vi "OEE_MAIN_set_default_reference.vi"(7 "all_config_info":T1, 8 "error_in":errorcluster, 11 "reference_selector":refnum<vi>) -> (0 "error_out":errorcluster, 3 "Default reference ok?":bool)   [LabVIEW 2019]
uses:
  ini/typedef/OEE_all_config_info.ctl
  ini/typedef/OEE_main_ini_file.ctl
  queues/typedef/OEE_queue_refnums.ctl
  queues/typedef/OEE_MAIN_queue_element.ctl
  OEE_MAIN_sequence_state.ctl
  queues/typedef/OEE_SCREEN_1_queue_element.ctl
  SCREEN_1/OEE_SCREEN_1_sequence_state.ctl
  queues/typedef/OEE_SCREEN_2_queue_element.ctl
  SCREEN_2/OEE_SCREEN_2_sequence_state.ctl
  queues/typedef/OEE_PULSE_queue_element.ctl
  PULSE/OEE_PULSE_sequence_state.ctl
  queues/typedef/OEE_GRAPH_TOGGLE_TIMER_queue_element.ctl
  SCREEN_2/GRAPH_TOGGLE_TIMER/OEE_GRAPH_TOGGLE_TIMER_sequence_state.ctl
  FGV/reference_selector/FGV_OEE_reference_selector.ctl
  _misc/AULocalize/SubVIs/Get Localized Phrase Compact Interface 0D.vi
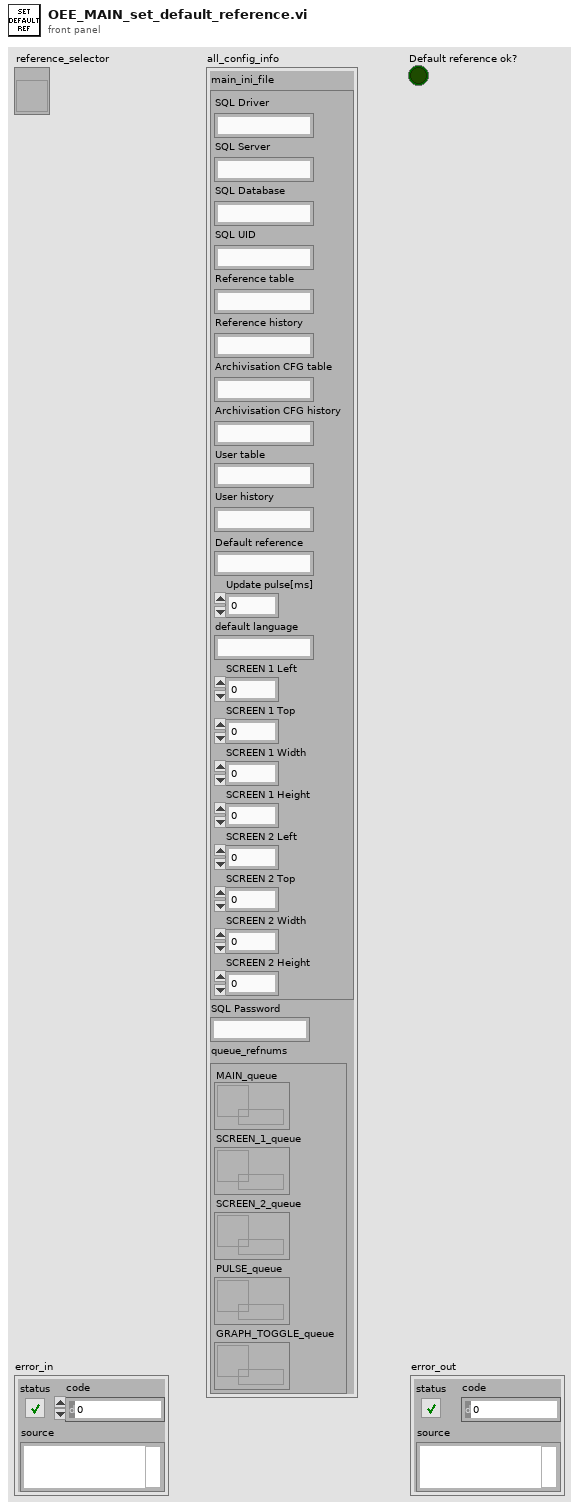
[diagram p1: front panel]
types:
  T1 = typedef "OEE_all_config_info.ctl" = cluster{"main_ini_file":T2, "SQL Password":string, "queue_refnums":T3}
  T2 = typedef "OEE_main_ini_file.ctl" = cluster{"SQL Driver":string, "SQL Server":string, "SQL Database":string, "SQL UID":string, "Reference table":string, "Reference history":string, "Archivisation CFG table":string, "Archivisation CFG history":string, "User table":string, "User history":string, "Default reference":string, "Update pulse[ms]":i32, "default language":string, "SCREEN 1 Left":i16, "SCREEN 1 Top":i16, "SCREEN 1 Width":i16, "SCREEN 1 Height":i16, "SCREEN 2 Left":i16, "SCREEN 2 Top":i16, "SCREEN 2 Width":i16, "SCREEN 2 Height":i16}
  T3 = typedef "OEE_queue_refnums.ctl" = cluster{"MAIN_queue":refnum<queue>, "SCREEN_1_queue":refnum<queue>, "SCREEN_2_queue":refnum<queue>, "PULSE_queue":refnum<queue>, "GRAPH_TOGGLE_queue":refnum<queue>}
  T4 = typedef "FGV_OEE_reference_selector.ctl" = enum16{"initialize", "set_values", "enable", "disable", "disable_gray", "get_reference_list", "get_active_reference"}
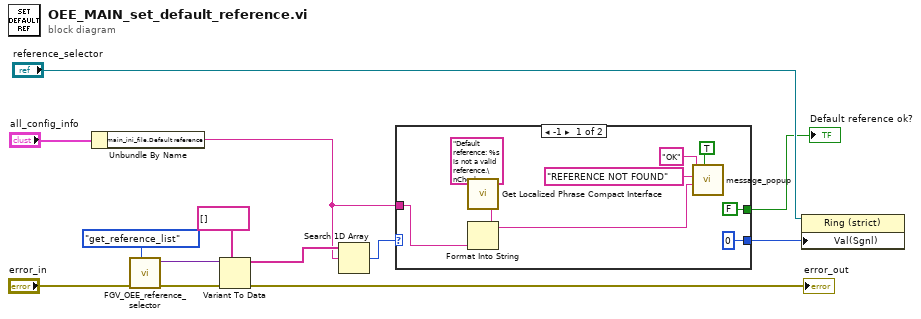
[diagram p0: block diagram]
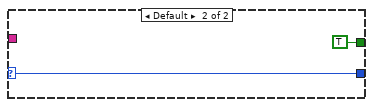
[diagram p2: hidden frame]
diagram:
  n1 = Unbundle By Name("all_config_info") -> ("main_ini_file.Default reference"=w5:string)
  n2 = call "FGV_OEE_reference_selector.vi"("options"=FGV_OEE_reference_selector."get_reference_list", "error_in"="error_in") -> ("error_out"=w11:errorcluster, "output"=w4:variant)  [unwired: 8 in]
  n3 = Variant To Data(error in=w11, type=string[] [], Variant=w4) -> (data=w7:string[], error out=→"error_out":errorcluster)
  n4 = Search 1D Array(1D array=w7, element=w5) -> (index of element=w6:i32)  [unwired: 1 in]
  n5 = case shown="-1" w6 {
    selector: w6 -> [_ w24]
    tunnel: w5 -> [w18 _]
    tunnel: [0 ("index of element") w24] -> w2
    tunnel: [FALSE TRUE] -> w1
    frame -1 {
      n6 = call-poly "Get Localized Phrase Compact Interface.vi"("Key"="Default reference: %s is not a valid reference.\nCheck reference definiton in database, change default reference in config file, or select another valid reference manually." ("format string")) -> ("Translated Phrase"=w14:string)
      n7 = Format Into String(format string=w14, w18) -> (resulting string=w19:string)  [unwired: 2 in, 1 out]
      n8 = call "message_popup.vi"("Warning(T)/Info(F)"=TRUE, "Message"=w19, "Title"="REFERENCE NOT FOUND", "Button Label"="OK") -> ()  [unwired: 7 in, 1 out]
    }
    frame Default {
    }
  }
  "Default reference ok?" <- w1
  n9 = property on="Property Node" class="Ring (strict)"(reference="reference_selector", "Val(Sgnl)"=w2) -> ()  [unwired: 1 in, 2 out]
